vi "delMN.vi"(0 "object in":refnum<class "interface.lvclass">, 1 "簇":cluster{"MN":string, "PW":string}={"MN"="平台数据发送系统", "PW"="平台数据发送系统"}, 5 "error in (no error)":errorcluster) -> (14 "object out":refnum<class "interface.lvclass">, 15 "删除标记":bool, 19 "error out":errorcluster)   [LabVIEW 2016, in "interface.lvclass"]
uses:
  interface.lvclass
  <vilib>/registry/registry.llb/Registry RtKey.ctl
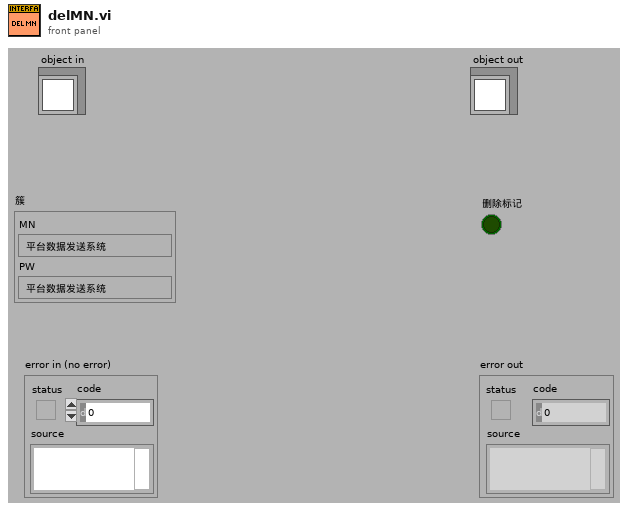
[diagram p1: front panel]
types:
  T1 = typedef "Registry RtKey.ctl" = enum32{"HKEY_CLASSES_ROOT", "HKEY_CURRENT_USER", "HKEY_LOCAL_MACHINE", "HKEY_USERS", "HKEY_PERFORMANCE_DATA", "HKEY_CURRENT_CONFIG", "HKEY_DYN_DATA"}
  T2 = typedef "Registry refnum.ctl" = refnum<k1>
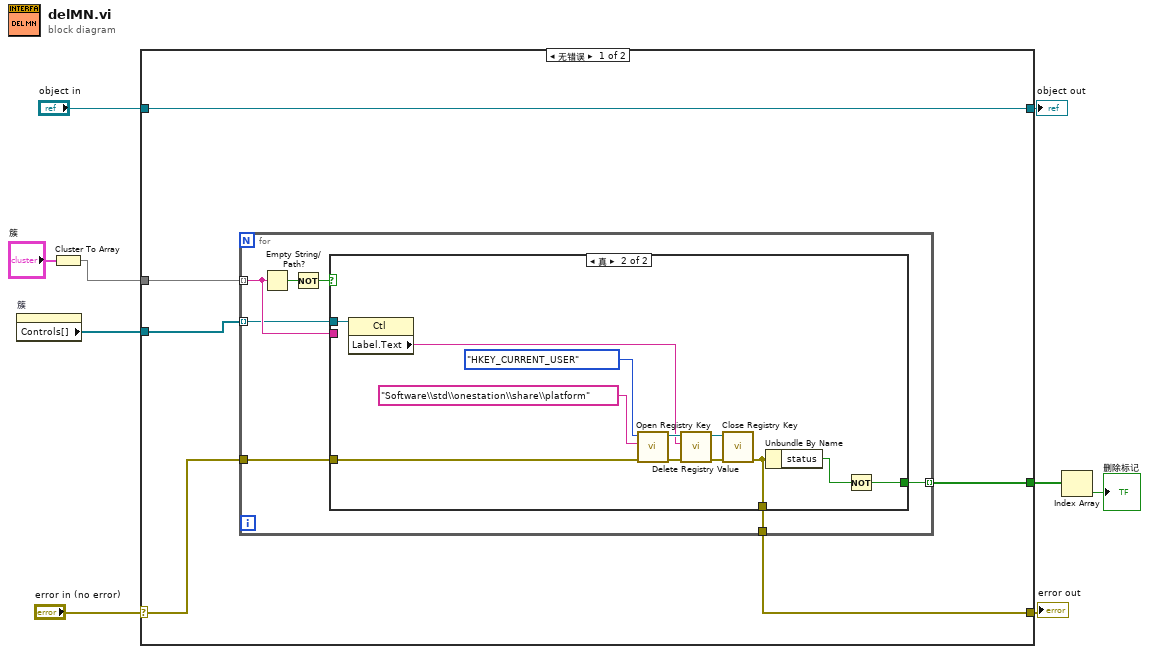
[diagram p0: block diagram]
diagram:
  n1 = property on="簇" class="Clust (严格)"() -> ("Controls[]"=w3:refnum<vi>[])  [unwired: 2 in, 2 out]
  n2 = Cluster To Array(cluster="簇") -> (array=w4:string[])
  n3 = case shown="无错误" "error in (no error)" {
    selector: "error in (no error)" -> [w14 w36]
    tunnel: [w13 w36] -> w8
    tunnel: [w15 w35] -> w6
    tunnel: "object in" -> [w15 w35]
    tunnel: w4 -> [w12 _]
    tunnel: w3 -> [w11 _]
    tunnel: [w10 _] -> w1
    frame No Error {
      n4 = for {
        tunnel: [w22] -> w10 mode=indexing
        tunnel: w12 -> [w19] mode=indexing
        tunnel: w11 -> [w18] mode=indexing
        tunnel: w14 -> [w17]
        tunnel: [w16] -> w13
        n5 = Empty String/Path?(string/path=w19) -> (empty?=w21:bool)
        n6 = Not(x=w21) -> (.not. x?=w20:bool)
        n7 = case shown="真" w20 {
          tunnel: w19 -> [_ _]
          tunnel: [_ w27] -> w22
          tunnel: w18 -> [_ w26]
          tunnel: w17 -> [_ w24]
          tunnel: [_ w23] -> w16
          frame False {
          }
          frame True {
            n8 = property class="Ctl"(reference=w26) -> ("Label.Text"=w25:string)  [unwired: 1 in, 2 out]
            n9 = call <vilib>:"Open Registry Key.vi"("error in (no error)"=w24, "subkey"="Software\\std\\onestation\\share\\platform", "root key (HKEY_LOCAL_MACHINE)"=Registry_RtKey."HKEY_CURRENT_USER") -> ("error out"=w30:errorcluster, "refnum out"=w32:T2)  [unwired: 7 in]
            n10 = call <vilib>:"Delete Registry Value.vi"("error in (no error)"=w30, "value"=w25, "refnum"=w32) -> ("error out"=w29:errorcluster, "refnum out"=w31:T2)  [unwired: 7 in]
            n11 = call <vilib>:"Close Registry Key.vi"("error in (no error)"=w29, "refnum"=w31) -> ("error out"=w23:errorcluster)  [unwired: 5 in]
            n12 = Unbundle By Name(w23) -> ("status"=w28:bool)
            n13 = Not(x=w28) -> (.not. x?=w27:bool)
          }
        }
      }
    }
    frame Error {
    }
  }
  "error out" <- w8
  "object out" <- w6
  n14 = Index Array(array=w1) -> (element=→"删除标记":bool)  [unwired: 1 in]
